vi "CalcChan.vi"(8 "Col":i32, 9 "Row":i32, 10 "Matrix":T1, 11 "Slot":i32) -> (2 "Chan":string, 3 "Matrix Chans":string)   [LabVIEW 2022 SP3, in "Switch_Keysight_34934A.lvlib" / "Switch_Keysight_34934A.lvclass"]
uses:
  Switch_Keysight_34934A.lvclass
  Matrix.ctl
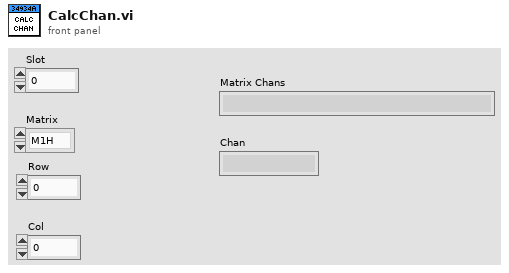
[diagram p1: front panel]
types:
  T1 = typedef "Switch_Keysight_34934A.lvlib/Switch_Keysight_34934A.lvclass/Matrix.ctl" = enum16{"M1H", "M2H", "M1L", "M2L"}
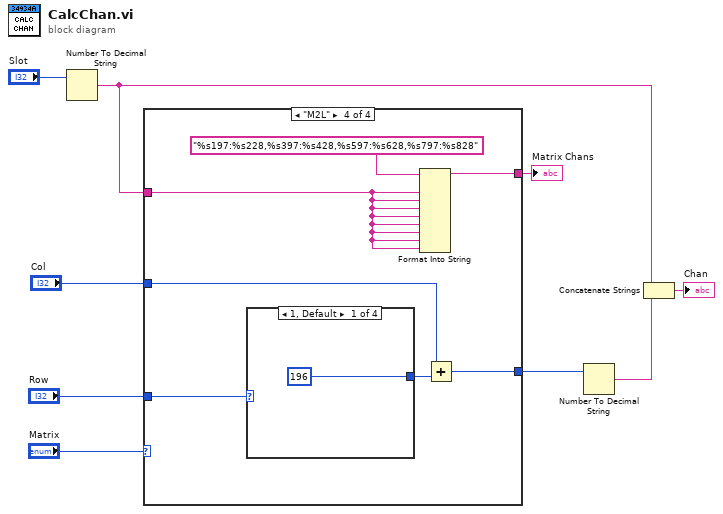
[diagram p0: block diagram]
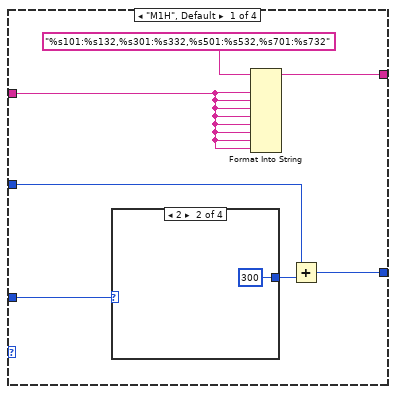
[diagram p2: hidden frame]
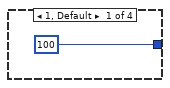
[diagram p3: hidden frame]
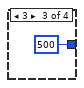
[diagram p4: hidden frame]
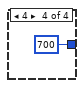
[diagram p5: hidden frame]
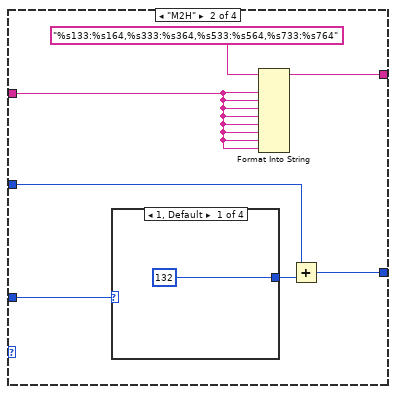
[diagram p6: hidden frame]
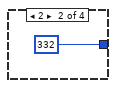
[diagram p7: hidden frame]
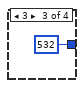
[diagram p8: hidden frame]
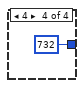
[diagram p9: hidden frame]
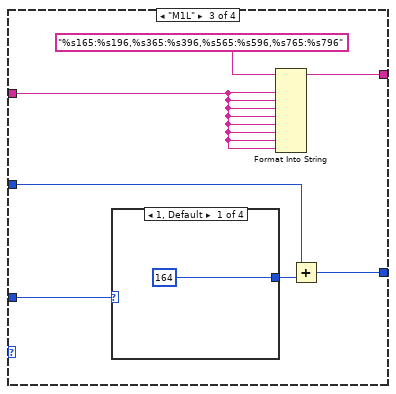
[diagram p10: hidden frame]
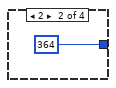
[diagram p11: hidden frame]
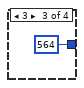
[diagram p12: hidden frame]
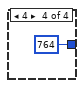
[diagram p13: hidden frame]
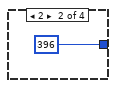
[diagram p14: hidden frame]
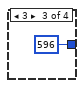
[diagram p15: hidden frame]
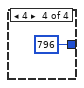
[diagram p16: hidden frame]
diagram:
  n1 = Number To Decimal String(number="Slot") -> (decimal integer string=w2:string)  [unwired: 1 in]
  n2 = case shown="\"M2L\"" "Matrix" {
    tunnel: "Row" -> [w16 w27 w38 w49]
    tunnel: "Col" -> [w14 w25 w36 w47]
    tunnel: [w13 w24 w35 w46] -> w6
    tunnel: w2 -> [w11 w22 w33 w44]
    tunnel: [w10 w21 w32 w43] -> w1
    frame "M1H", Default {
      n3 = case shown="2" w16 {
        tunnel: [100 300 500 700] -> w15
        frame 1, Default {
        }
        frame 2 {
        }
        frame 3 {
        }
        frame 4 {
        }
      }
      n4 = Format Into String(format string="%s101:%s132,%s301:%s332,%s501:%s532,%s701:%s732", w11, w11, w11, w11, w11, w11, w11, w11) -> (resulting string=w10:string)  [unwired: 2 in, 1 out]
      n5 = Add(x=w14, y=w15) -> (x+y=w13:i32)
    }
    frame "M2H" {
      n6 = case shown="1, Default" w27 {
        tunnel: [132 332 532 732] -> w26
        frame 1, Default {
        }
        frame 2 {
        }
        frame 3 {
        }
        frame 4 {
        }
      }
      n7 = Format Into String(format string="%s133:%s164,%s333:%s364,%s533:%s564,%s733:%s764", w22, w22, w22, w22, w22, w22, w22, w22) -> (resulting string=w21:string)  [unwired: 2 in, 1 out]
      n8 = Add(x=w25, y=w26) -> (x+y=w24:i32)
    }
    frame "M1L" {
      n9 = case shown="1, Default" w38 {
        tunnel: [164 364 564 764] -> w37
        frame 1, Default {
        }
        frame 2 {
        }
        frame 3 {
        }
        frame 4 {
        }
      }
      n10 = Format Into String(format string="%s165:%s196,%s365:%s396,%s565:%s596,%s765:%s796", w33, w33, w33, w33, w33, w33, w33, w33) -> (resulting string=w32:string)  [unwired: 2 in, 1 out]
      n11 = Add(x=w36, y=w37) -> (x+y=w35:i32)
    }
    frame "M2L" {
      n12 = case shown="1, Default" w49 {
        tunnel: [196 396 596 796] -> w48
        frame 1, Default {
        }
        frame 2 {
        }
        frame 3 {
        }
        frame 4 {
        }
      }
      n13 = Format Into String(format string="%s197:%s228,%s397:%s428,%s597:%s628,%s797:%s828", w44, w44, w44, w44, w44, w44, w44, w44) -> (resulting string=w43:string)  [unwired: 2 in, 1 out]
      n14 = Add(x=w47, y=w48) -> (x+y=w46:i32)
    }
  }
  "Matrix Chans" <- w1
  n15 = Number To Decimal String(number=w6) -> (decimal integer string=w4:string)  [unwired: 1 in]
  n16 = Concatenate Strings(w2, w4) -> (→"Chan":string)
